vi "Close.vi"(8 "error in (no error)":errorcluster, 10 "skvc in":string[][](array[string]), 11 "Ini Path in":path) -> (0 "error out":errorcluster, 3 "Ini Path out":path)   [LabVIEW 2018, in "Config.lvlib"]
uses:
  Config.lvlib
  <vilib>/ErrorRing/Error Ring.xnode
  <vilib>/Utility/error.llb/Error Cluster From Error Code.vi
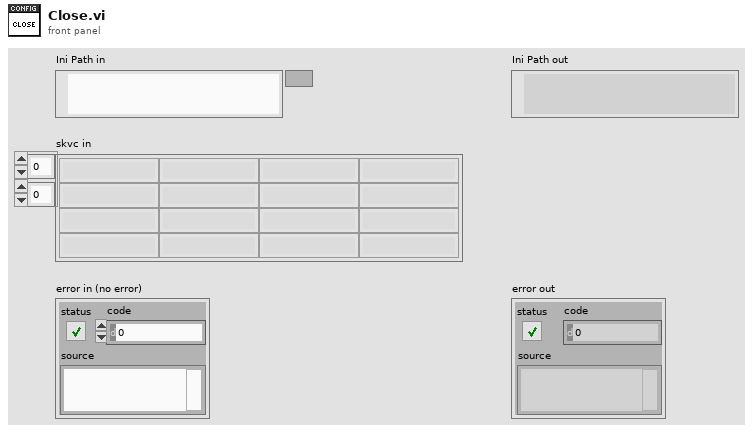
[diagram p1: front panel]
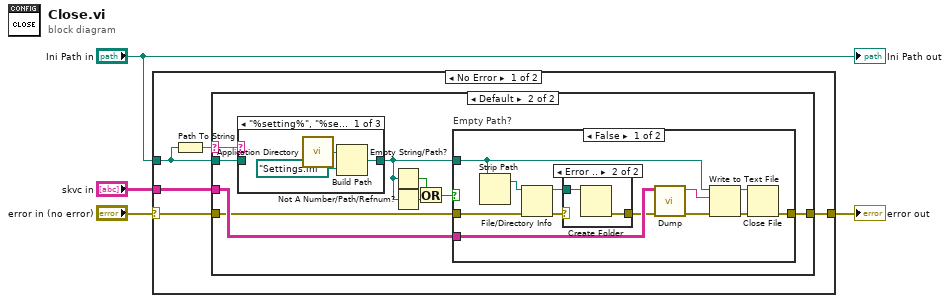
[diagram p0: block diagram]
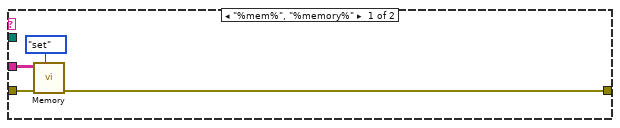
[diagram p2: hidden frame]
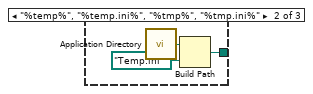
[diagram p3: hidden frame]
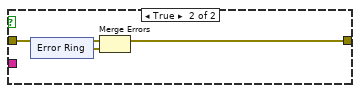
[diagram p6: hidden frame]
diagram:
  n1 = case shown="No Error" "error in (no error)" {
    selector: "error in (no error)" -> [w8 w52]
    tunnel: [w9 w52] -> w4
    tunnel: "Ini Path in" -> [w6 _]
    tunnel: "skvc in" -> [w5 _]
    frame No Error {
      n2 = Path To String(path=w6) -> (string=w7:string)
      n3 = case shown="Default" w7 {
        selector: w7 -> [_ w15]
        tunnel: [w12 w20] -> w9
        tunnel: w8 -> [w11 w18]
        tunnel: w6 -> [_ w16]
        tunnel: w5 -> [w10 w19]
        frame "%mem%", "%memory%" {
          n4 = call "Memory.vi"("Action (get)"=enum8{"get", "set"}."set", "error in (no error)"=w11, "skvc in"=w10) -> ("error out"=w12:errorcluster)  [unwired: 7 in, 1 out]
        }
        frame Default {
          n5 = case shown="\"%setting%\", \"%setting.ini%\", \"%settings%\", \"%settings.ini%\"" w15 {
            tunnel: w16 -> [_ _ w29]
            tunnel: [w25 w28 w29] -> w14
            frame "%setting%", "%setting.ini%", "%settings%", "%settings.ini%" {
              n6 = call <vilib>:"Application Directory.vi"() -> ("Application Directory"=w24:path)
              n7 = Build Path(base path=w24, name or relative path=path "Settings.ini") -> (appended path=w25:path)
            }
            frame "%temp%", "%temp.ini%", "%tmp%", "%tmp.ini%" {
              n8 = call <vilib>:"Application Directory.vi"() -> ("Application Directory"=w27:path)
              n9 = Build Path(base path=w27, name or relative path=path "Temp.ini") -> (appended path=w28:path)
            }
            frame Default {
            }
          }
          n10 = Empty String/Path?(string/path=w14) -> (empty?=w21:bool)
          n11 = Not A Number/Path/Refnum?(number/path/refnum=w14) -> (NaN/Path/Refnum?=w22:bool)
          n12 = Or(x=w21, y=w22) -> (x .or. y?=w17:bool)
          n13 = case "Empty Path?" shown="False" w17 {
            tunnel: [w30 w45] -> w20
            tunnel: w19 -> [w38 _]
            tunnel: w18 -> [w33 w46]
            tunnel: w14 -> [w31 _]
            frame False {
              n14 = Strip Path(path=w31) -> (stripped path=w35:path)  [unwired: 1 out]
              n15 = File/Directory Info(path=w35, error in=w33) -> (path out=w34:path, error out=w36:errorcluster)  [unwired: 5 out]
              n16 = case shown="Error .." w36 {
                selector: w36 -> [w42 _]
                tunnel: [w42 w44] -> w32
                tunnel: w34 -> [_ w43]
                frame No Error {
                }
                frame Error {
                  n17 = Create Folder(path (use dialog)=w43) -> (error out=w44:errorcluster)  [unwired: 2 in, 2 out]
                }
              }
              n18 = call "Dump.vi"("error in (no error)"=w32, "skvc"=w38) -> ("error out"=w39:errorcluster, "Text"=w37:string)  [unwired: 8 in]
              n19 = Write to Text File(file (use dialog)=w31, text=w37, error in=w39) -> (refnum out=w40:refnum<file>, error out=w41:errorcluster)  [unwired: 1 in, 1 out]
              n20 = Close File(refnum=w40, error in=w41) -> (error out=w30:errorcluster)  [unwired: 1 out]
            }
            frame True {
              n21 = xnode "Error Ring"() -> ("error out"=w47:errorcluster)
              n22 = Merge Errors(w46, w47) -> (w45:errorcluster)
            }
          }
        }
      }
    }
    frame Error {
    }
  }
  "error out" <- w4
  "Ini Path out" <- "Ini Path in"
